vi "Material-ChoosePart#-Spec.vi"(8 "error in (no error)":errorcluster, 11 "Material-RunTest.lvclass":refnum<class "Material-RunTest.lvclass">) -> (0 "error out":errorcluster, 1 "Cancel Test":bool, 2 "Invalid Spec Values":bool, 3 "Material-RunTest.lvclass out":refnum<class "Material-RunTest.lvclass">)   [LabVIEW 2013, in "Material-RunTest.lvclass"]
uses:
  Material-RunTest.lvclass
  Material-RunTest.lvclass/Material-RunTest.ctl
  <vilib>/addons/database/Connection.llb/DB Tools Open Connec (Path).vi
  <userlib>/_OpenG.lib/array/array.llb/Search 1D Array (String)__ogtk.vi
  <userlib>/_OpenG.lib/array/array.llb/Delete Elements from 1D Array (String)__ogtk.vi
  <userlib>/_OpenG.lib/array/array.llb/Empty 2D Array (String)__ogtk.vi
  <vilib>/Utility/error.llb/Error Cluster From Error Code.vi
  <vilib>/ErrorRing/Error Ring.xnode
  <vilib>/addons/database/NI_Database_API.lvlib
panel:
  in  "Lot Number":string
  in  "Cancel Test":bool
  in  "Choose Part":bool
  out "ZMaximum Thickness":dbl format="%_5g"
  out "ZMinimum Thickness":dbl format="%_5g"
  out "ZNominal Thickness":dbl format="%_5g"
  in  "Part Number to Search For":string
  in  "Cancel Search":bool
  in  "Search Button":bool
  in  "Part Numbers":i32(listbox)
  # "Please Enter Lot Number"
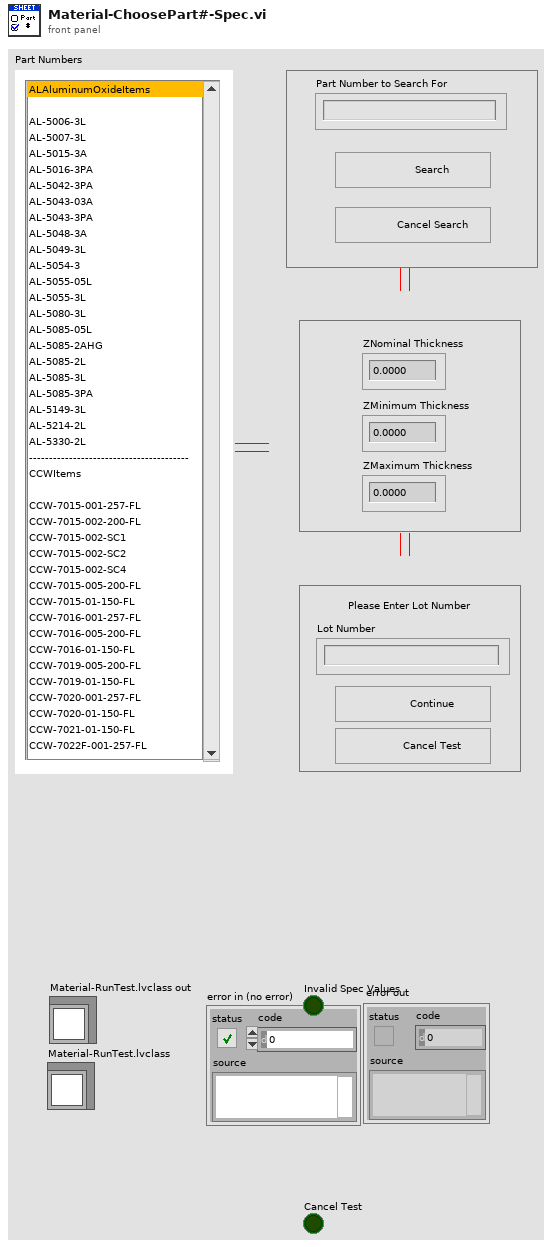
[diagram p1: front panel]
types:
  T1 = typedef "NI_Database_API.lvlib/Conn ObjectReference.ctl" = refnum<k1>
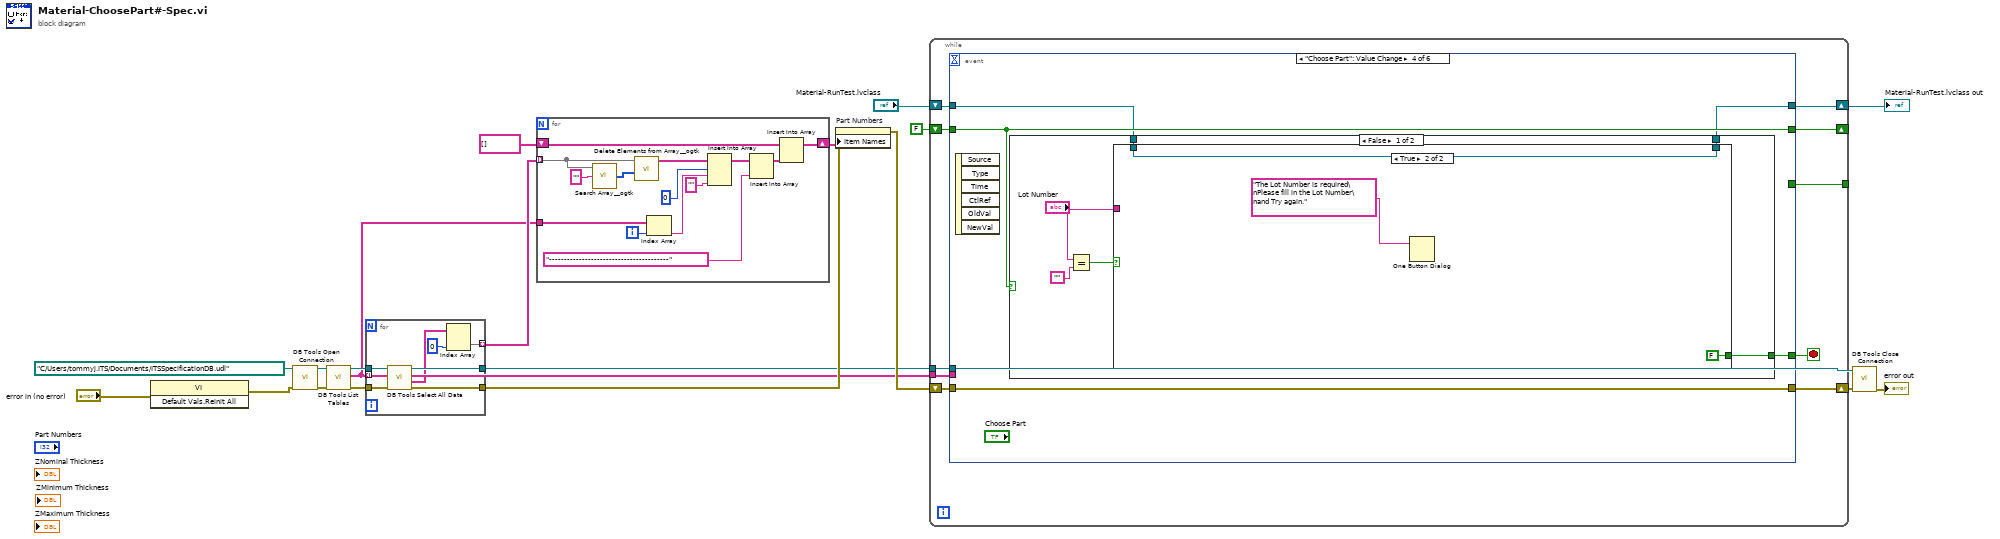
[diagram p0: block diagram]
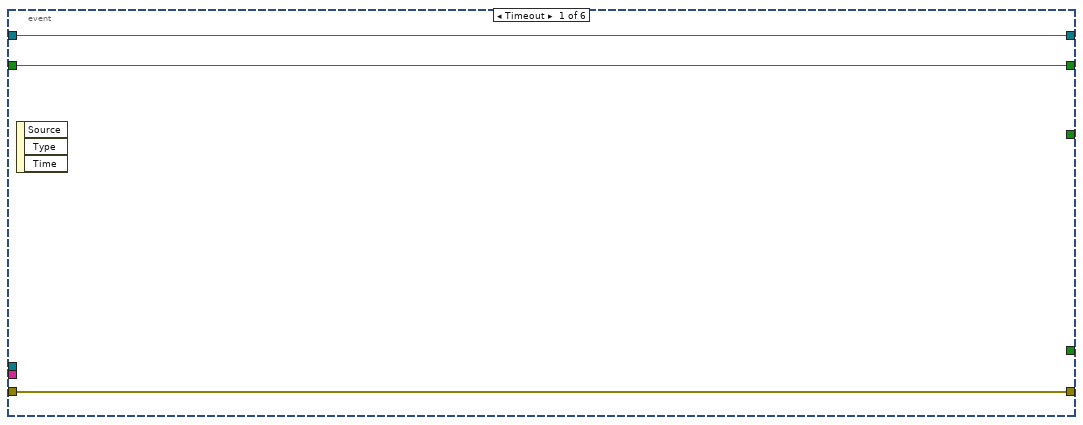
[diagram p2: hidden frame]
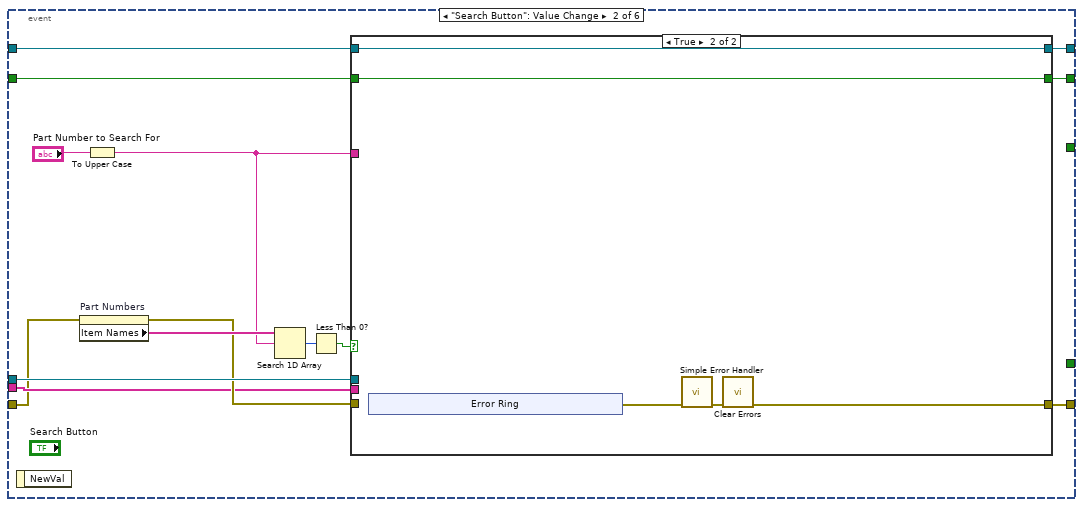
[diagram p3: hidden frame]
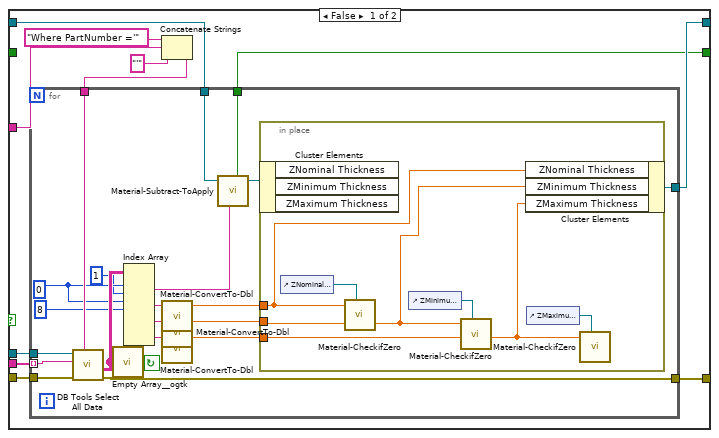
[diagram p4: hidden frame]
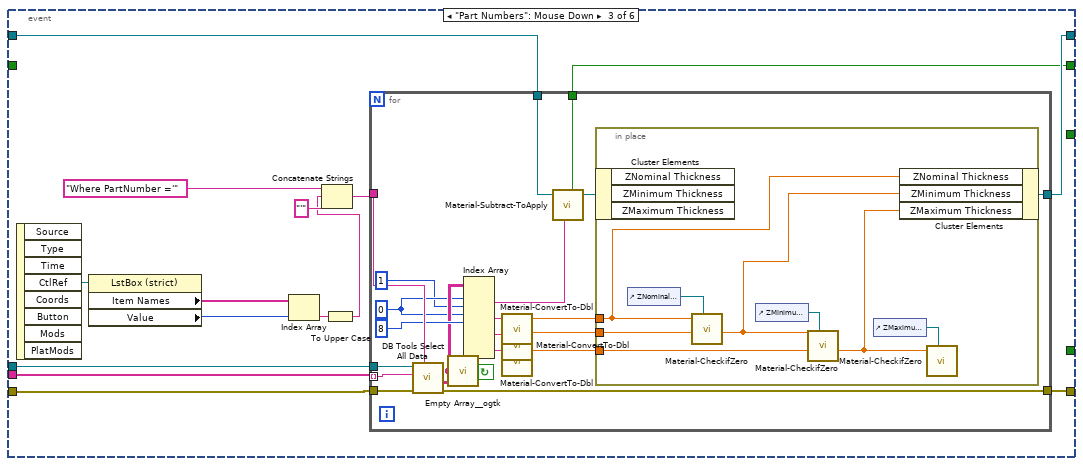
[diagram p5: hidden frame]
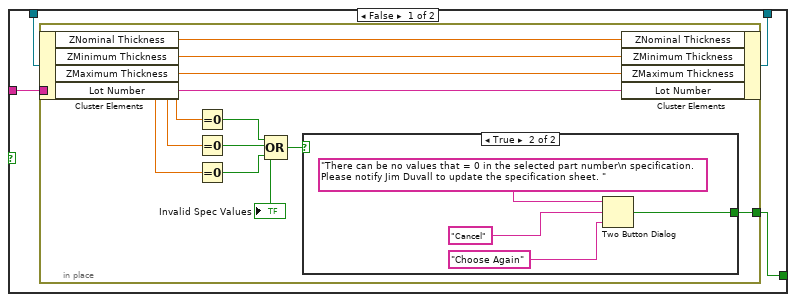
[diagram p6: hidden frame]
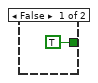
[diagram p7: hidden frame]
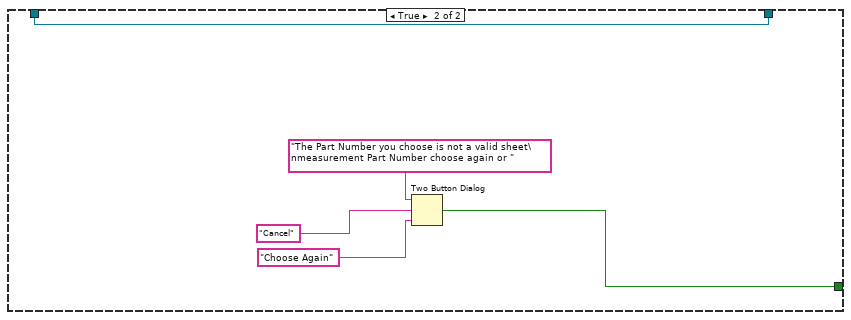
[diagram p8: hidden frame]
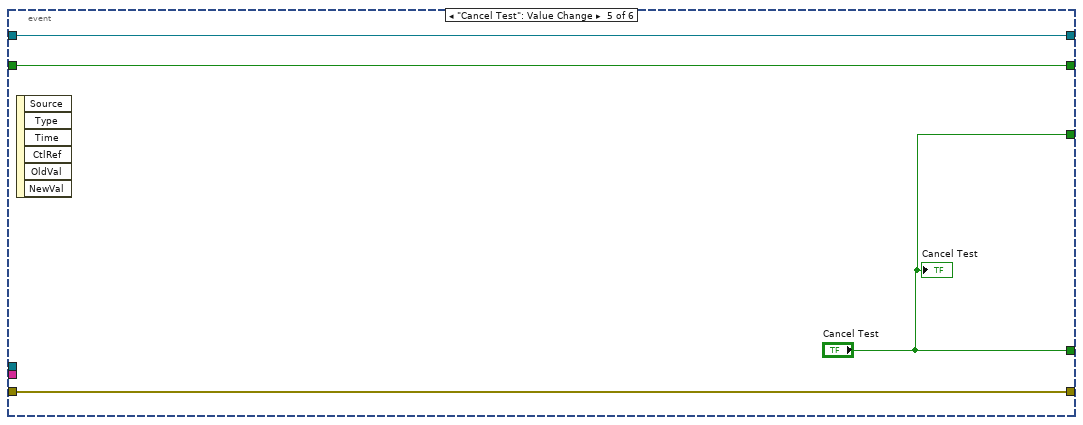
[diagram p9: hidden frame]
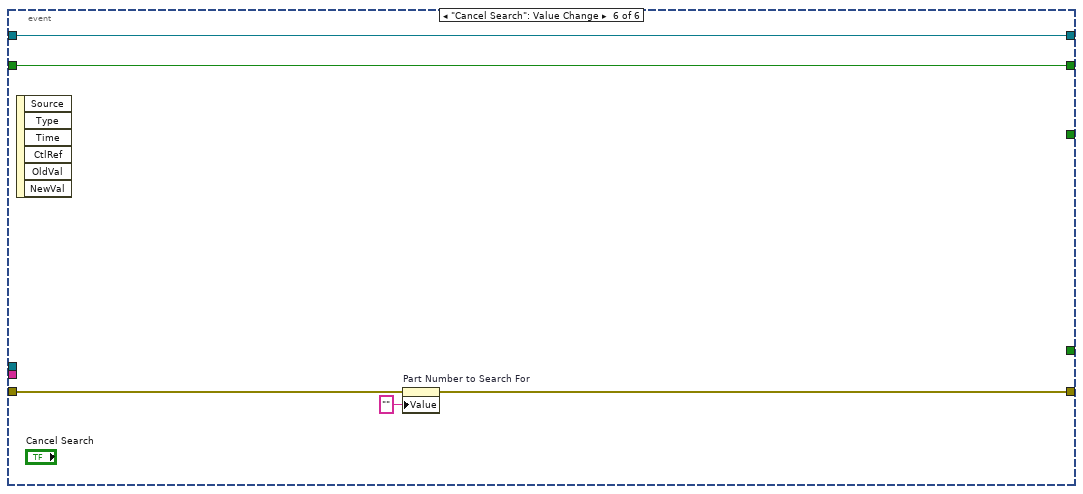
[diagram p10: hidden frame]
diagram:
  n1 = invoke class="VI" method="Default Vals.Reinit All"(error in="error in (no error)") -> (error out=w8:errorcluster)  [unwired: 2 in, 2 out]
  n2 = call-poly <vilib>:"DB Tools Open Connection.vi"("error in (no error)"=w8, "connection information"=path "C:/Users/tommyj.ITS/Documents/ITSSpecificationDB.udl") -> ("error out"=w18:errorcluster, "connection reference"=w17:T1)  [unwired: 6 in]
  n3 = call <vilib>:"DB Tools List Tables.vi"("error in (no error)"=w18, "connection reference"=w17) -> ("error out"=w15:errorcluster, "tables"=w9:string[], "connection reference out"=w16:T1)  [unwired: 3 in]
  n4 = for {
    tunnel: w9 -> [w26] mode=indexing
    tunnel: w16 -> [w25]
    tunnel: w15 -> [w27]
    tunnel: [w20] -> w13 mode=indexing
    tunnel: [w24] -> w7
    tunnel: [w23] -> w10
    n5 = call <vilib>:"DB Tools Select All Data.vi"("error in (no error)"=w27, "table"=w26, "connection reference"=w25) -> ("error out"=w23:errorcluster, "data"=w22:string[][], "connection reference out"=w24:T1)  [unwired: 3 in]
    n6 = Index Array(array=w22, index (col)=0 ("disabled index (col)")) -> (element=w20:string[])  [unwired: 1 in]
  }
  n7 = for {
    tunnel: w13 -> [w35] mode=indexing
    shift-right: [w41] -> w12
    shift-left: string[] [] -> [w40]
    tunnel: w9 -> [w32]
    i -> [w31]
    n8 = call-poly <userlib>:"Search Array__ogtk.vi"("Array"=w35, "Element Data"="") -> ("Indices of Elements"=w36:i32[])  [unwired: 7 in]
    n9 = call-poly <userlib>:"Delete Elements from Array__ogtk.vi"("indices"=w36, "array"=w35) -> ("array w/ subset deleted"=w34:string[])  [unwired: 8 in, 1 out]
    n10 = Index Array(array=w32, index=w31) -> (element=w30:string)
    n11 = Insert Into Array(array=w34, index=0, new element #1=w30, new element #2="" ("new element/subarray")) -> (w29:string[])
    n12 = Insert Into Array(array=w29, new element="----------------------------------------" ("new element/subarray")) -> (w38:string[])  [unwired: 1 in]
    n13 = Insert Into Array(array=w40, new element=w38) -> (w41:string[])  [unwired: 1 in]
  }
  n14 = property on="Part Numbers" class="LstBox (strict)"(error in=w10, "Item Names"=w12) -> (error out=w11:errorcluster)  [unwired: 1 in, 1 out]
  n15 = while {
    tunnel: w7 -> [w51]
    tunnel: w9 -> [w50]
    shift-right: [w49] -> w2
    shift-left: w11 -> [w48]
    tunnel: [w44] -> _
    shift-right: [w43] -> _
    shift-left: FALSE ("Part Number no Valid for sheet") -> [w42]
    shift-right: [w45] -> w3
    shift-left: "Material-RunTest.lvclass" -> [w46]
    stop <- w47 stop-if-true
    n16 = event shown="[3] \"Choose Part\": Value Change" {
      selector: _ -> [_ _ _ _ _ _]
      dyn-events: _ -> [_ _ _ _ _ _]
      timeout: _ -> [_ _ _ _ _ _]
      tunnel: w51 -> [_ w64 w123 _ _ _]
      tunnel: w50 -> [_ w62 w121 _ _ _]
      tunnel: [w54 w61 w120 w163 w199 w203] -> w49
      tunnel: w48 -> [w54 w59 w122 w163 w199 w204]
      tunnel: [_ _ _ w161 "Cancel Test" _] -> w47
      tunnel: w46 -> [w53 w58 w119 w160 w198 w201]
      tunnel: [w53 w57 w118 w159 w198 w201] -> w45
      tunnel: [_ _ _ _ "Cancel Test" _] -> w44
      tunnel: [w52 w56 w117 w162 w196 w200] -> w43
      tunnel: w42 -> [w52 w55 _ w162 w196 w200]
      event Timeout {
        n17 = event-data() -> ()  [unwired: 1 in, 3 out]
      }
      event "Search Button": Value Change {
        n18 = event-data() -> ()  [unwired: 1 in, 1 out]
        n19 = property on="Part Numbers" class="LstBox (strict)"(error in=w59) -> (error out=w63:errorcluster, "Item Names"=w68:string[])  [unwired: 1 in, 1 out]
        n20 = To Upper Case(1:"Part Number to Search For") -> (0:w60:string)
        n21 = Search 1D Array(1D array=w68, element=w60) -> (index of element=w67:i32)  [unwired: 1 in]
        n22 = Less Than 0?(x=w67) -> (x < 0?=w65:bool)
        n23 = case shown="True" w65 {
          tunnel: w64 -> [w78 _]
          tunnel: w63 -> [w79 _]
          tunnel: w62 -> [w77 _]
          tunnel: [w72 w109] -> w61
          tunnel: w60 -> [w75 _]
          tunnel: w58 -> [w71 w108]
          tunnel: [w70 w108] -> w57
          tunnel: [w69 w107] -> w56
          tunnel: w55 -> [_ w107]
          frame False {
            n24 = Concatenate Strings("Where PartNumber ='" ("optional clause"), w75, "'" ("string")) -> (w73:string)
            n25 = for {
              tunnel: w79 -> [w100]
              tunnel: w78 -> [w99]
              tunnel: w73 -> [w98]
              tunnel: w77 -> [w97] mode=indexing
              tunnel: [w90] -> w72
              tunnel: w71 -> [w83]
              tunnel: [w89] -> w70
              tunnel: [w80] -> w69
              stop <- w96 continue-if-true
              w85 = 0 ("disabled index (row)")
              n26 = call <vilib>:"DB Tools Select All Data.vi"("optional clause"=w98, "error in (no error)"=w100, "table"=w97, "connection reference"=w99) -> ("error out"=w90:errorcluster, "data"=w95:string[][])  [unwired: 2 in, 1 out]
              n27 = call-poly <userlib>:"Empty Array__ogtk.vi"("Array"=w95) -> ("Empty Array?"=w96:bool)  [unwired: 8 in]
              n28 = Index Array(array=w95, index (row) #1=w85, index (col) #1=1 ("disabled index (col)"), index (row) #2=w85, index (col) #2=8 ("disabled index (col)")) -> (element #1=w81:string, element #2=w93:string, element #3=w92:string, element #4=w91:string)  [unwired: 4 in]
              n29 = call "Material-ConvertTo-Dbl.vi"("DBL String"=w93) -> ("DBL liner out"=w88:dbl)  [unwired: 8 in]
              n30 = call "Material-ConvertTo-Dbl.vi"("DBL String"=w92) -> ("DBL liner out"=w87:dbl)  [unwired: 8 in]
              n31 = call "Material-ConvertTo-Dbl.vi"("DBL String"=w91) -> ("DBL liner out"=w86:dbl)  [unwired: 8 in]
              n32 = call "Material-Subtract-ToApply.vi"("Material-RunTest in"=w83, "Description"=w81) -> ("Part Number no Valid for sheet"=w80:bool, "Material-RunTest out"=w82:refnum<class "Material-RunTest.lvclass">)  [unwired: 6 in]
              n33 = in-place {
                in-place-border: w88 -> [w105]
                in-place-border: w87 -> [w103]
                in-place-border: w86 -> [w102]
                n34 = in-place-cluster #1(w82) -> ()  [unwired: 3 out]
                n35 = control-ref of="ZNominal Thickness"() -> (w106:refnum<vi>)
                n36 = call "Material-CheckifZero.vi"("DBL liner in"=w105, "Digital in"=w106) -> ()  [unwired: 9 in]
                n37 = control-ref of="ZMinimum Thickness"() -> (w104:refnum<vi>)
                n38 = call "Material-CheckifZero.vi"("DBL liner in"=w103, "Digital in"=w104) -> ()  [unwired: 9 in]
                n39 = in-place-cluster #1("ZNominal Thickness"=w105, "ZMinimum Thickness"=w103, "ZMaximum Thickness"=w102) -> (w89:refnum<class "Material-RunTest.lvclass">)
                n40 = control-ref of="ZMaximum Thickness"() -> (w101:refnum<vi>)
                n41 = call "Material-CheckifZero.vi"("DBL liner in"=w102, "Digital in"=w101) -> ()  [unwired: 9 in]
              }
            }
          }
          frame True {
            n42 = xnode "Error Ring"() -> ("error out"=w111:errorcluster)
            n43 = call <vilib>:"Simple Error Handler.vi"("error in (no error)"=w111) -> ("error out"=w110:errorcluster)  [unwired: 4 in, 4 out]
            n44 = call <vilib>:"Clear Errors.vi"("error in (no error)"=w110) -> ("error out"=w109:errorcluster)  [unwired: 6 in]
          }
        }
      }
      event "Part Numbers": Mouse Down {
        n45 = event-data() -> ("CtlRef"=w131:refnum<vi>)  [unwired: 1 in, 7 out]
        n46 = property class="LstBox (strict)"(reference=w131) -> ("Item Names"=w130:string[], "Value"=w129:i32)  [unwired: 1 in, 2 out]
        n47 = Index Array(array=w130, index=w129) -> (element=w125:string)
        n48 = To Upper Case(1:w125) -> (0:w124:string)
        n49 = Concatenate Strings("Where PartNumber ='" ("optional clause"), w124, "'" ("string")) -> (w126:string)
        n50 = for {
          tunnel: w122 -> [w152]
          tunnel: w123 -> [w151]
          tunnel: w126 -> [w150]
          tunnel: w121 -> [w149] mode=indexing
          tunnel: [w143] -> w120
          tunnel: w119 -> [w134]
          tunnel: [w142] -> w118
          tunnel: [w132] -> w117
          stop <- w148 continue-if-true
          w137 = 0 ("disabled index (row)")
          n51 = call <vilib>:"DB Tools Select All Data.vi"("optional clause"=w150, "error in (no error)"=w152, "table"=w149, "connection reference"=w151) -> ("error out"=w143:errorcluster, "data"=w138:string[][])  [unwired: 2 in, 1 out]
          n52 = call-poly <userlib>:"Empty Array__ogtk.vi"("Array"=w138) -> ("Empty Array?"=w148:bool)  [unwired: 8 in]
          n53 = Index Array(array=w138, index (row) #1=w137, index (col) #1=1 ("disabled index (row)"), index (row) #2=w137, index (col) #2=8 ("disabled index (col)")) -> (element #1=w133:string, element #2=w146:string, element #3=w145:string, element #4=w144:string)  [unwired: 4 in]
          n54 = call "Material-ConvertTo-Dbl.vi"("DBL String"=w146) -> ("DBL liner out"=w141:dbl)  [unwired: 8 in]
          n55 = call "Material-ConvertTo-Dbl.vi"("DBL String"=w145) -> ("DBL liner out"=w140:dbl)  [unwired: 8 in]
          n56 = call "Material-ConvertTo-Dbl.vi"("DBL String"=w144) -> ("DBL liner out"=w139:dbl)  [unwired: 8 in]
          n57 = call "Material-Subtract-ToApply.vi"("Material-RunTest in"=w134, "Description"=w133) -> ("Part Number no Valid for sheet"=w132:bool, "Material-RunTest out"=w135:refnum<class "Material-RunTest.lvclass">)  [unwired: 6 in]
          n58 = in-place {
            in-place-border: w141 -> [w155]
            in-place-border: w140 -> [w154]
            in-place-border: w139 -> [w153]
            n59 = in-place-cluster #2(w135) -> ()  [unwired: 3 out]
            n60 = control-ref of="ZNominal Thickness"() -> (w158:refnum<vi>)
            n61 = call "Material-CheckifZero.vi"("DBL liner in"=w155, "Digital in"=w158) -> ()  [unwired: 9 in]
            n62 = control-ref of="ZMinimum Thickness"() -> (w157:refnum<vi>)
            n63 = call "Material-CheckifZero.vi"("DBL liner in"=w154, "Digital in"=w157) -> ()  [unwired: 9 in]
            n64 = control-ref of="ZMaximum Thickness"() -> (w156:refnum<vi>)
            n65 = in-place-cluster #2("ZNominal Thickness"=w155, "ZMinimum Thickness"=w154, "ZMaximum Thickness"=w153) -> (w142:refnum<class "Material-RunTest.lvclass">)
            n66 = call "Material-CheckifZero.vi"("DBL liner in"=w153, "Digital in"=w156) -> ()  [unwired: 9 in]
          }
        }
      }
      event "Choose Part": Value Change {
        n67 = event-data() -> ()  [unwired: 1 in, 6 out]
        n68 = case shown="False" w162 {
          tunnel: [w167 w194] -> w161
          tunnel: w160 -> [w169 w191]
          tunnel: [w168 w191] -> w159
          frame False {
            n69 = Equal?(x="Lot Number", y="") -> (x = y?=w165:bool)
            n70 = case shown="True" w165 {
              tunnel: w169 -> [w173 w188]
              tunnel: [w172 w188] -> w168
              tunnel: [w171 FALSE ("T button?")] -> w167
              tunnel: "Lot Number" -> [w170 _]
              frame False {
                n71 = in-place {
                  in-place-border: [w175] -> w171
                  in-place-border: w170 -> [w174]
                  n72 = in-place-cluster #3(w173) -> ("ZNominal Thickness"=w182:dbl, "ZMinimum Thickness"=w181:dbl, "ZMaximum Thickness"=w180:dbl)  [unwired: 1 out]
                  n73 = Equal To 0?(x=w182) -> (x = 0?=w179:bool)
                  n74 = Equal To 0?(x=w181) -> (x = 0?=w178:bool)
                  n75 = Equal To 0?(x=w180) -> (x = 0?=w177:bool)
                  n76 = Compound Arithmetic op=OR(w179, w178, w177) -> (w176:bool)
                  "Invalid Spec Values" <- w176
                  n77 = case shown="True" w176 {
                    tunnel: [TRUE ("T button?") w184] -> w175
                    frame False {
                    }
                    frame True {
                      n78 = Two Button Dialog(message="There can be no values that = 0 in the selected part number\n specification. Please notify Jim Duvall to update the specification sheet. " ("T button name (\"OK\")"), 1:"Choose Again" ("T button name (\"OK\")"), 2:"Cancel" ("F button name (\"Cancel\")")) -> (T button?=w184:bool)
                    }
                  }
                  n79 = in-place-cluster #3("ZNominal Thickness"=w182, "ZMinimum Thickness"=w181, "ZMaximum Thickness"=w180, "Lot Number"=w174) -> (w172:refnum<class "Material-RunTest.lvclass">)
                }
              }
              frame True {
                n80 = One Button Dialog(message="The Lot Number is required\nPlease fill in the Lot Number\nand Try again.") -> ()  [unwired: 1 in, 1 out]
              }
            }
          }
          frame True {
            n81 = Two Button Dialog(message="The Part Number you choose is not a valid sheet\nmeasurement Part Number choose again or ", 1:"Choose Again" ("T button name (\"OK\")"), 2:"Cancel" ("F button name (\"Cancel\")")) -> (T button?=w194:bool)
          }
        }
      }
      event "Cancel Test": Value Change {
        n82 = event-data() -> ()  [unwired: 1 in, 6 out]
        "Cancel Test" <- "Cancel Test"
      }
      event "Cancel Search": Value Change {
        n83 = event-data() -> ()  [unwired: 1 in, 6 out]
        n84 = property on="Part Number to Search For" class="Str"(error in=w204, "Value"="" ("Part Number to Search For")) -> (error out=w203:errorcluster)  [unwired: 1 in, 1 out]
      }
    }
  }
  "Material-RunTest.lvclass out" <- w3
  n85 = call <vilib>:"DB Tools Close Connection.vi"("error in (no error)"=w2, "connection reference"=w7) -> ("error out"=→"error out":errorcluster)  [unwired: 5 in]
